vi "New - GetStuff.vi"() -> ()   [LabVIEW 2017]
uses:
  typedefs/Asset Info.ctl
  typedefs/Sensor Info.ctl
  typedefs/Metric Info.ctl
  <vilib>/addons/InsightCM/MessageBus/MessageService/IcmMessageService.lvclass
panel:
  out "error out":errorcluster
  out "Array":T1[](array[typedef])
  in  "stop":bool
  in  "Get assets":bool
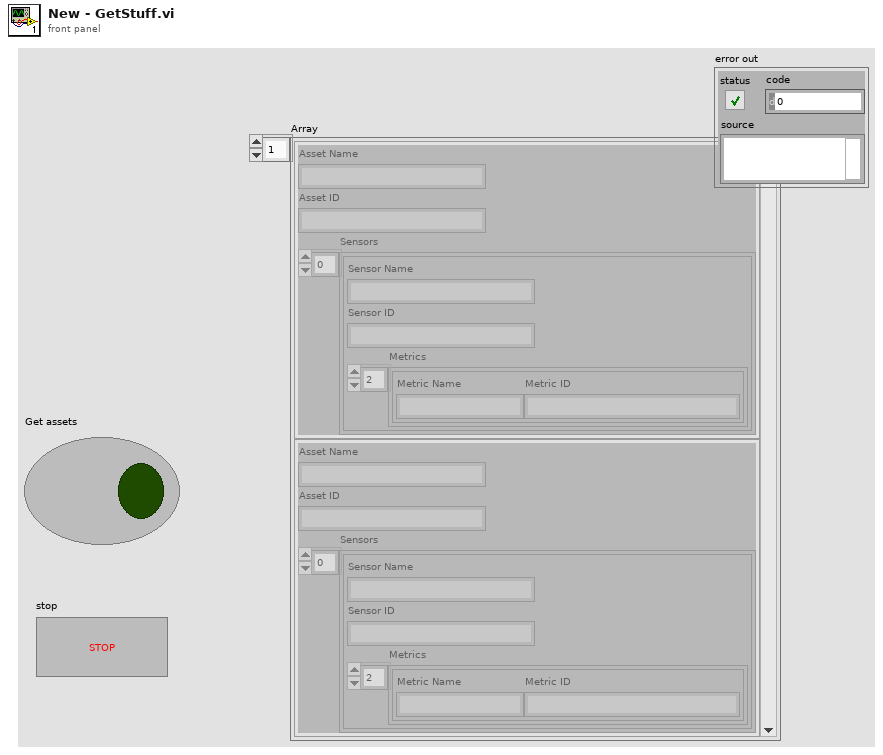
[diagram p1: front panel]
types:
  T1 = typedef "Asset Info.ctl" = cluster{"Asset Name":string, "Asset ID":string, "Sensors":T2[]}
  T2 = typedef "Sensor Info.ctl" = cluster{"Sensor Name":string, "Sensor ID":string, "Metrics":T3[]}
  T3 = typedef "Metric Info.ctl" = cluster{"Metric Name ":string, "Metric ID":string}
  T4 = typedef "AssetNodeView.ctl" = cluster{"Id":string, "Type":string, "Name":string, "ParentIds":string[], "State":T5, "MeasType":string, "Metrics":T6[], "References":T8[], "HasOperatingStates":bool}
  T5 = typedef "AssetState.ctl" = cluster{"Disabled":bool}
  T6 = typedef "Metric.ctl" = cluster{"Id":string, "Name":string, "Unit":string, "Properties":T7[], "MetricDefinitionInstanceId":string}
  T7 = typedef "KeyValuePair.ctl" = cluster{"Key":string, "Value":string}
  T8 = typedef "AssetNodeReference.ctl" = cluster{"NodeId":string, "Name":string}
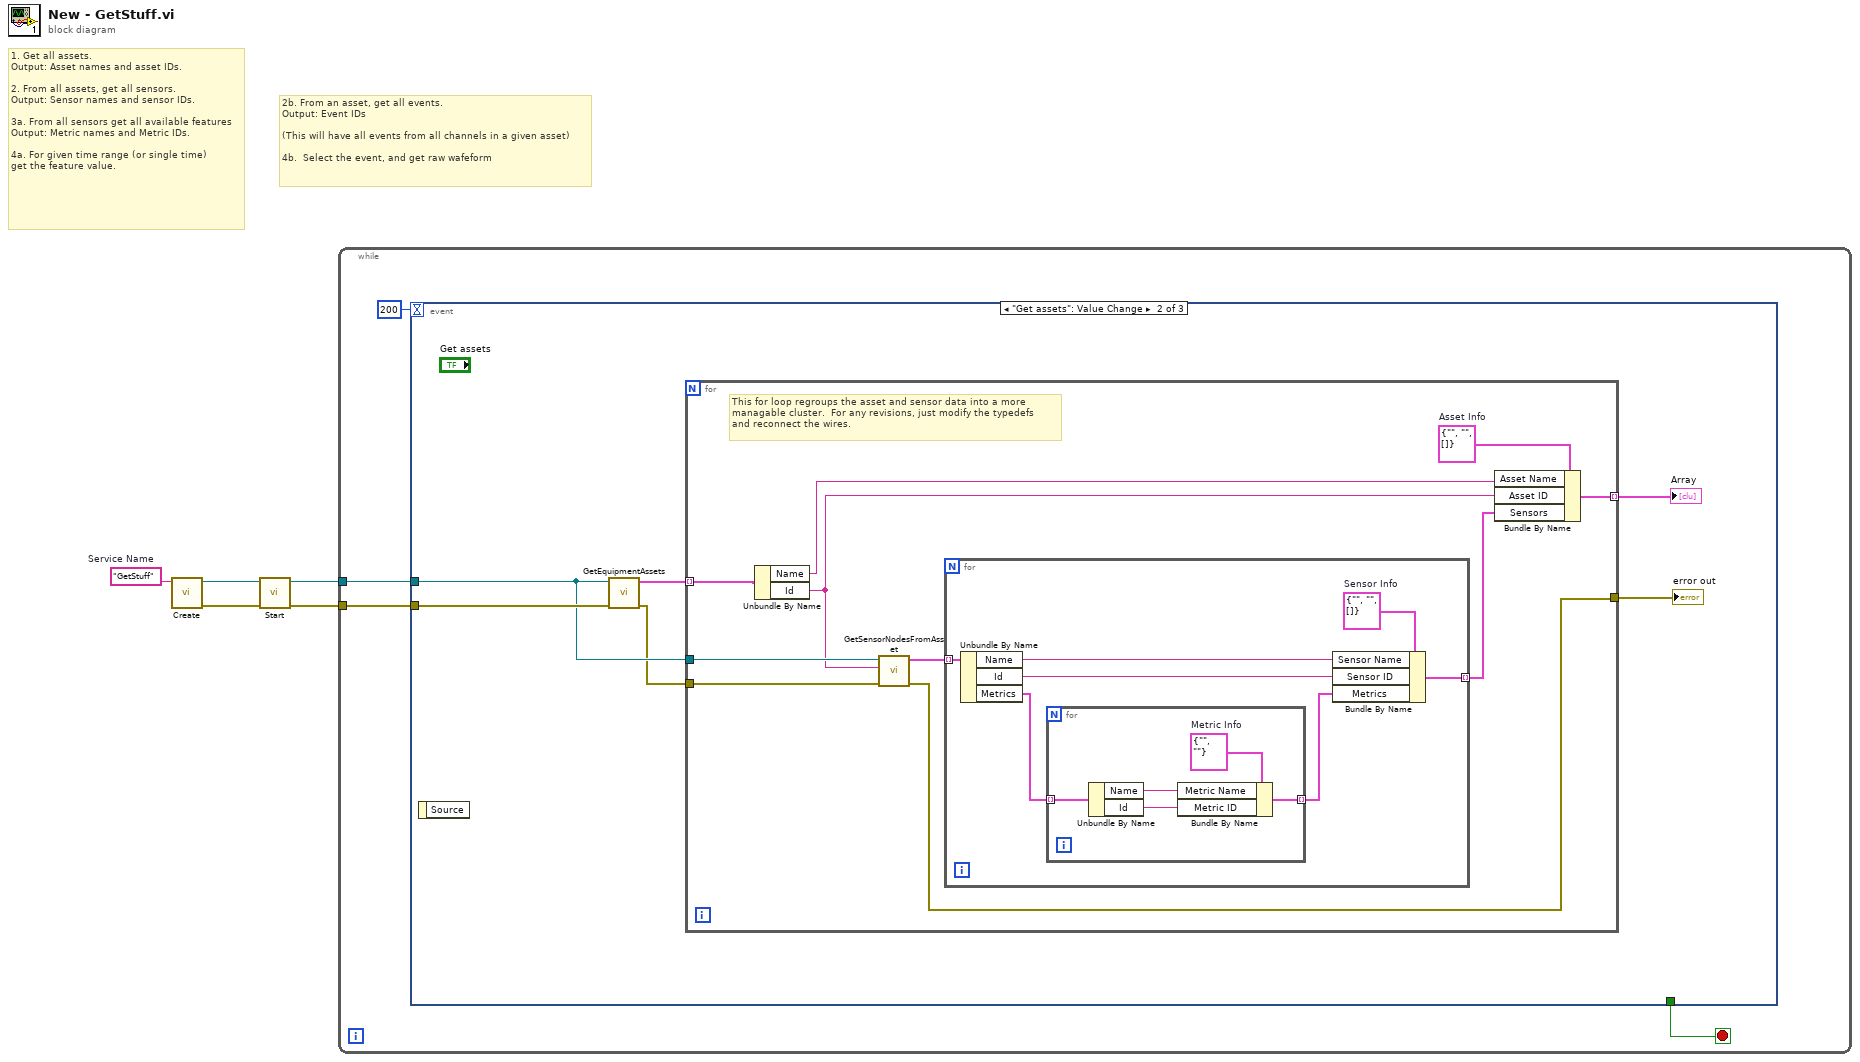
[diagram p0: block diagram]
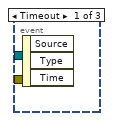
[diagram p2: hidden frame]
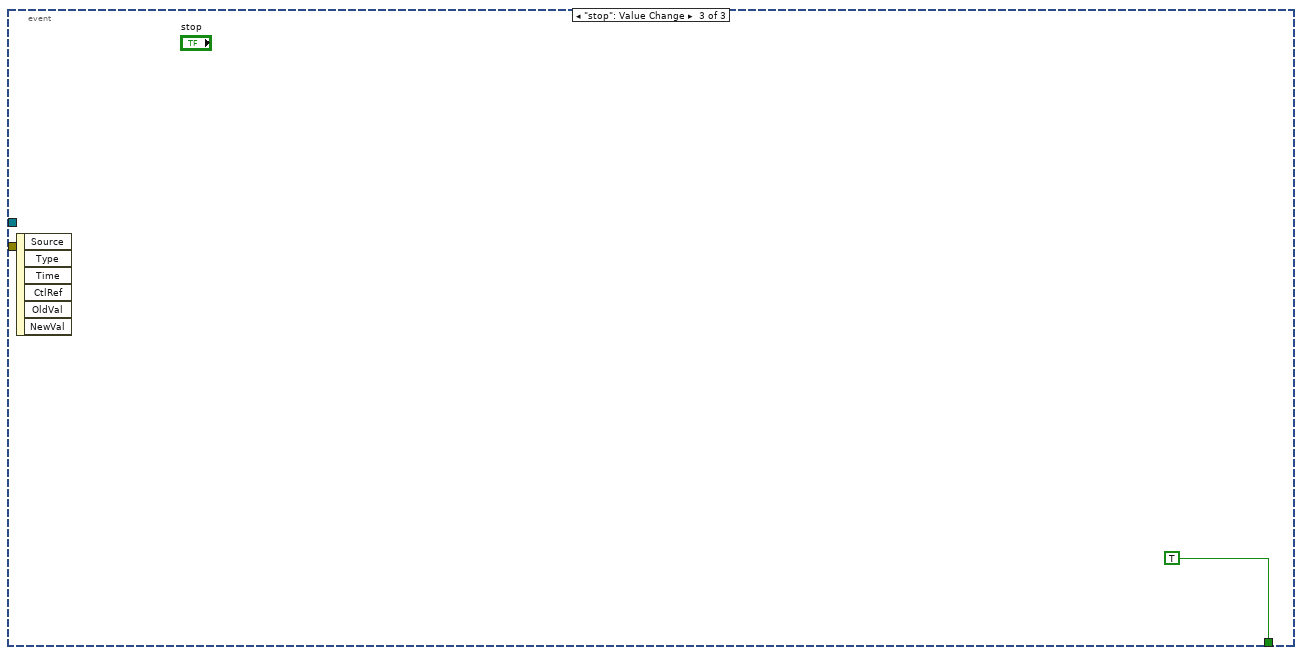
[diagram p3: hidden frame]
diagram:
  w5 = "GetStuff"  # Service Name
  # "2b. From an asset, get all events.\nOutput: Event IDs\n\n(This will have all events from all channels in a given asset)\n\n4b.  Select the event, and get raw wafeform"
  # "1. Get all assets.  \nOutput: Asset names and asset IDs.\n\n2. From all assets, get all sensors.\nOutput: Sensor names and sensor IDs.\n\n3a. From all sensors get all available features\nOutput: Metric names and Metric IDs.\n\n4a. For given time range (or single time)\nget the feature value."
  n1 = call <vilib>:"Create.vi"("service name"=w5) -> ("error out"=w3:errorcluster, "service out"=w4:refnum<class "IcmMessageService.lvclass">)  [unwired: 9 in]
  n2 = call <vilib>:"Start.vi"("error in (no error)"=w3, "service in"=w4) -> ("error out"=w1:errorcluster, "service out"=w2:refnum<class "IcmMessageService.lvclass">)  [unwired: 8 in]
  n3 = while {
    tunnel: w2 -> [w6]
    tunnel: w1 -> [w7]
    stop <- w9 stop-if-true
    n4 = event shown="[1] \"Get assets\": Value Change" {
      selector: _ -> [_ _ _]
      dyn-events: _ -> [_ _ _]
      timeout: 200 -> [_ _ _]
      tunnel: [_ _ TRUE] -> w9
      tunnel: w6 -> [_ w13 _]
      tunnel: w7 -> [_ w15 _]
      event Timeout {
        n5 = event-data() -> ()  [unwired: 1 in, 3 out]
      }
      event "Get assets": Value Change {
        n6 = event-data() -> ()  [unwired: 1 in, 1 out]
        n7 = call "GetEquipmentAssets.vi"("error in (no error)"=w15, "service"=w13) -> ("error out"=w12:errorcluster, "AssetNodes"=w14:T4[])  [unwired: 8 in]
        n8 = for {
          tunnel: w14 -> [w25] mode=indexing
          tunnel: w13 -> [w24]
          tunnel: w12 -> [w23]
          tunnel: [w17] -> w11 mode=indexing
          tunnel: [w16] -> w10
          w22 = T1 {"Asset Name"="", "Asset ID"="", "Sensors"=[]}  # Asset Info
          # "This for loop regroups the asset and sensor data into a more \nmanagable cluster.  For any revisions, just modify the typedefs\nand reconnect the wires."
          n9 = Unbundle By Name(w25) -> ("Name"=w21:string, "Id"=w20:string)
          n10 = call "GetSensorNodesFromAsset.vi"("error in (no error)"=w23, "Asset ID"=w20, "ICM Service in"=w24) -> ("error out"=w16:errorcluster, "SensorNodes"=w19:T4[])  [unwired: 7 in]
          n11 = for {
            tunnel: w19 -> [w32] mode=indexing
            tunnel: [w26] -> w18 mode=indexing
            w31 = T2 {"Sensor Name"="", "Sensor ID"="", "Metrics"=[]}  # Sensor Info
            n12 = Unbundle By Name(w32) -> ("Name"=w30:string, "Id"=w29:string, "Metrics"=w28:T6[])
            n13 = for {
              tunnel: w28 -> [w36] mode=indexing
              tunnel: [w33] -> w27 mode=indexing
              w37 = T3 {"Metric Name "="", "Metric ID"=""}  # Metric Info
              n14 = Unbundle By Name(w36) -> ("Name"=w35:string, "Id"=w34:string)
              n15 = Bundle By Name(cluster=w37, "Metric Name"=w35, "Metric ID"=w34) -> (w33:T3)
            }
            n16 = Bundle By Name(cluster=w31, "Sensor Name"=w30, "Sensor ID"=w29, "Metrics"=w27) -> (w26:T2)
          }
          n17 = Bundle By Name(cluster=w22, "Asset Name"=w21, "Asset ID"=w20, "Sensors"=w18) -> (w17:T1)
        }
        "Array" <- w11
        "error out" <- w10
      }
      event "stop": Value Change {
        n18 = event-data() -> ()  [unwired: 1 in, 6 out]
      }
    }
  }
